vi "SMSD_cmd_Data_format.vi"(10 "DATA (0)":u32 format="%x", 11 "COMMAND (END)":T1(ring)) -> (3 "SMSD_CMD_out":u8[](array[numeric]))   [LabVIEW 2021, in "SMSD.lvclass"]
uses:
  SMSD.lvclass
  Data Unit/SMSD Data Unit/SMSD_CMD_Type.ctl
  Data Unit/SMSD Data Unit/SMSD Data Unit.lvclass
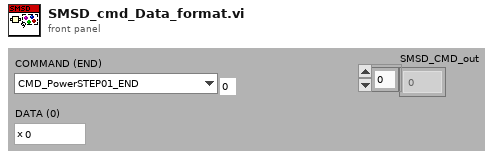
[diagram p1: front panel]
types:
  T1 = enum8{"CMD_PowerSTEP01_END", "CMD_PowerSTEP01_GET_SPEED", "CMD_PowerSTEP01_STATUS_IN_EVENT", "CMD_PowerSTEP01_SET_MODE", "CMD_PowerSTEP01_GET_MODE", "CMD_PowerSTEP01_SET_MIN_SPEED", "CMD_PowerSTEP01_SET_MAX_SPEED", "CMD_PowerSTEP01_SET_ACC", "CMD_PowerSTEP01_SET_DEC", "CMD_PowerSTEP01_SET_FS_SPEED", "CMD_PowerSTEP01_SET_MASK_EVENT", "CMD_PowerSTEP01_GET_ABS_POS", "CMD_PowerSTEP01_GET_EL_POS", "CMD_PowerSTEP01_GET_STATUS_AND_CLR", "CMD_PowerSTEP01_RUN_F", "CMD_PowerSTEP01_RUN_R", "CMD_PowerSTEP01_MOVE_F", "CMD_PowerSTEP01_MOVE_R", "CMD_PowerSTEP01_GO_TO_F", "CMD_PowerSTEP01_GO_TO_R", "CMD_PowerSTEP01_GO_UNTIL_F", "CMD_PowerSTEP01_GO_UNTIL_R", "CMD_PowerSTEP01_SCAN_ZERO_F", "CMD_PowerSTEP01_SCAN_ZERO_R", "CMD_PowerSTEP01_SCAN_LABEL_F", "CMD_PowerSTEP01_SCAN_LABEL_R", "CMD_PowerSTEP01_GO_ZERO", "CMD_PowerSTEP01_GO_LABEL", "CMD_PowerSTEP01_GO_TO", "CMD_PowerSTEP01_RESET_POS", "CMD_PowerSTEP01_RESET_POWERSTEP01", "CMD_PowerSTEP01_SOFT_STOP", "CMD_PowerSTEP01_HARD_STOP", "CMD_PowerSTEP01_SOFT_HI_Z", "CMD_PowerSTEP01_HARD_HI_Z", "CMD_PowerSTEP01_SET_WAIT", "CMD_PowerSTEP01_SET_RELE", "CMD_PowerSTEP01_CLR_RELE", "CMD_PowerSTEP01_GET_RELE", "CMD_PowerSTEP01_WAIT_IN0", "CMD_PowerSTEP01_WAIT_IN1", "CMD_PowerSTEP01_GOTO_PROGRAM", "CMD_PowerSTEP01_GOTO_PROGRAM_IF_IN0", "CMD_PowerSTEP01_GOTO_PROGRAM_IF_IN1", "CMD_PowerSTEP01_LOOP_PROGRAM", "CMD_PowerSTEP01_CALL_PROGRAM", "CMD_PowerSTEP01_RETURN_PROGRAM", "CMD_PowerSTEP01_START_PROGRAM_MEM0", "CMD_PowerSTEP01_START_PROGRAM_MEM1", "CMD_PowerSTEP01_START_PROGRAM_MEM2", "CMD_PowerSTEP01_START_PROGRAM_MEM3", "CMD_PowerSTEP01_STOP_PROGRAM_MEM", "CMD_PowerSTEP01_STEP_CLOCK", "CMD_PowerSTEP01_STOP_USB", "CMD_PowerSTEP01_GET_MIN_SPEED", "CMD_PowerSTEP01_GET_MAX_SPEED", "CMD_PowerSTEP01_GET_STACK", "CMD_PowerSTEP01_GOTO_PROGRAM_IF_ZERO", "CMD_PowerSTEP01_GOTO_PROGRAM_IF_IN_ZERO", "CMD_PowerSTEP01_WAIT_CONTINUE", "CMD_PowerSTEP01_SET_WAIT_2", "CMD_PowerSTEP01_SCAN_MARK2_F", "CMD_PowerSTEP01_SCAN_MARK2_R"}
  T2 = typedef "SMSD Data Unit.lvclass/SMSD_CMD_Type.ctl" = cluster{"RESERVE":u32, "ACTION":u32, "COMMAND":enum8{"CMD_PowerSTEP01_END", "CMD_PowerSTEP01_GET_SPEED", "CMD_PowerSTEP01_STATUS_IN_EVENT", "CMD_PowerSTEP01_SET_MODE", "CMD_PowerSTEP01_GET_MODE", "CMD_PowerSTEP01_SET_MIN_SPEED", "CMD_PowerSTEP01_SET_MAX_SPEED", "CMD_PowerSTEP01_SET_ACC", "CMD_PowerSTEP01_SET_DEC", "CMD_PowerSTEP01_SET_FS_SPEED", "CMD_PowerSTEP01_SET_MASK_EVENT", "CMD_PowerSTEP01_GET_ABS_POS", "CMD_PowerSTEP01_GET_EL_POS", "CMD_PowerSTEP01_GET_STATUS_AND_CLR", "CMD_PowerSTEP01_RUN_F", "CMD_PowerSTEP01_RUN_R", "CMD_PowerSTEP01_MOVE_F", "CMD_PowerSTEP01_MOVE_R", "CMD_PowerSTEP01_GO_TO_F", "CMD_PowerSTEP01_GO_TO_R", "CMD_PowerSTEP01_GO_UNTIL_F", "CMD_PowerSTEP01_GO_UNTIL_R", "CMD_PowerSTEP01_SCAN_ZERO_F", "CMD_PowerSTEP01_SCAN_ZERO_R", "CMD_PowerSTEP01_SCAN_LABEL_F", "CMD_PowerSTEP01_SCAN_LABEL_R", "CMD_PowerSTEP01_GO_ZERO", "CMD_PowerSTEP01_GO_LABEL", "CMD_PowerSTEP01_GO_TO", "CMD_PowerSTEP01_RESET_POS", "CMD_PowerSTEP01_RESET_POWERSTEP01", "CMD_PowerSTEP01_SOFT_STOP", "CMD_PowerSTEP01_HARD_STOP", "CMD_PowerSTEP01_SOFT_HI_Z", "CMD_PowerSTEP01_HARD_HI_Z", "CMD_PowerSTEP01_SET_WAIT", "CMD_PowerSTEP01_SET_RELE", "CMD_PowerSTEP01_CLR_RELE", "CMD_PowerSTEP01_GET_RELE", "CMD_PowerSTEP01_WAIT_IN0", "CMD_PowerSTEP01_WAIT_IN1", "CMD_PowerSTEP01_GOTO_PROGRAM", "CMD_PowerSTEP01_GOTO_PROGRAM_IF_IN0", "CMD_PowerSTEP01_GOTO_PROGRAM_IF_IN1", "CMD_PowerSTEP01_LOOP_PROGRAM", "CMD_PowerSTEP01_CALL_PROGRAM", "CMD_PowerSTEP01_RETURN_PROGRAM", "CMD_PowerSTEP01_START_PROGRAM_MEM0", "CMD_PowerSTEP01_START_PROGRAM_MEM1", "CMD_PowerSTEP01_START_PROGRAM_MEM2", "CMD_PowerSTEP01_START_PROGRAM_MEM3", "CMD_PowerSTEP01_STOP_PROGRAM_MEM", "CMD_PowerSTEP01_STEP_CLOCK", "CMD_PowerSTEP01_STOP_USB", "CMD_PowerSTEP01_GET_MIN_SPEED", "CMD_PowerSTEP01_GET_MAX_SPEED", "CMD_PowerSTEP01_GET_STACK", "CMD_PowerSTEP01_GOTO_PROGRAM_IF_ZERO", "CMD_PowerSTEP01_GOTO_PROGRAM_IF_IN_ZERO", "CMD_PowerSTEP01_WAIT_CONTINUE", "CMD_PowerSTEP01_SET_WAIT_2", "CMD_PowerSTEP01_SCAN_MARK2_F", "CMD_PowerSTEP01_SCAN_MARK2_R"}, "DATA":u32}
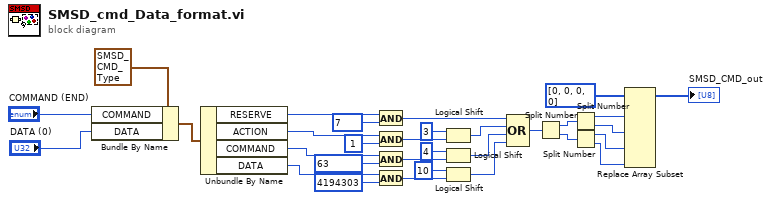
[diagram p0: block diagram]
diagram:
  n1 = Bundle By Name(cluster=T2 {"RESERVE"=0, "ACTION"=0, "COMMAND"=enum."CMD_PowerSTEP01_SOFT_STOP", "DATA"=0} ("SMSD_CMD"), "COMMAND"="COMMAND (END)", "DATA"="DATA (0)") -> (w1:T2)
  n2 = Unbundle By Name(w1) -> ("RESERVE"=w25:u32, "ACTION"=w21:u32, "COMMAND"=w19:T1, "DATA"=w15:u32)
  n3 = And(x=w25, y=u32 7) -> (x .and. y?=w23:u32)
  n4 = And(x=w21, y=u32 1) -> (x .and. y?=w18:u32)
  n5 = And(x=w19, y=u32 63) -> (x .and. y?=w17:u32)
  n6 = And(x=w15, y=u32 4194303) -> (x .and. y?=w14:u32)
  n7 = Logical Shift(y=i16 3, x=w18) -> (x << y=w28:u32)
  n8 = Logical Shift(y=i16 4, x=w17) -> (x << y=w27:u32)
  n9 = Logical Shift(y=i16 10, x=w14) -> (x << y=w26:u32)
  n10 = Compound Arithmetic op=OR(w23, w28, w27, w26) -> (w13:u32)
  n11 = Split Number(x=w13) -> (hi(x)=w12:u16, lo(x)=w11:u16)
  n12 = Split Number(x=w12) -> (hi(x)=w9:u8, lo(x)=w8:u8)
  n13 = Split Number(x=w11) -> (hi(x)=w7:u8, lo(x)=w6:u8)
  n14 = Replace Array Subset(array=u8[] [0, 0, 0, 0], new element #1=w9, new element #2=w8, new element #3=w7, new element #4=w6) -> (→"SMSD_CMD_out":u8[])  [unwired: 4 in]
